vi "Emballage mail expedition.vi"(1 "Tableau mail expedition":string[][](array[string]), 2 "Article":string) -> (0 "Email expedition":string)   [LabVIEW 2020]
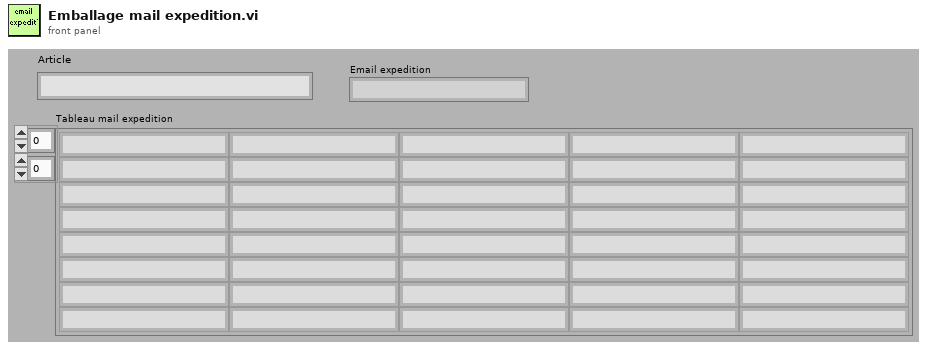
[diagram p1: front panel]
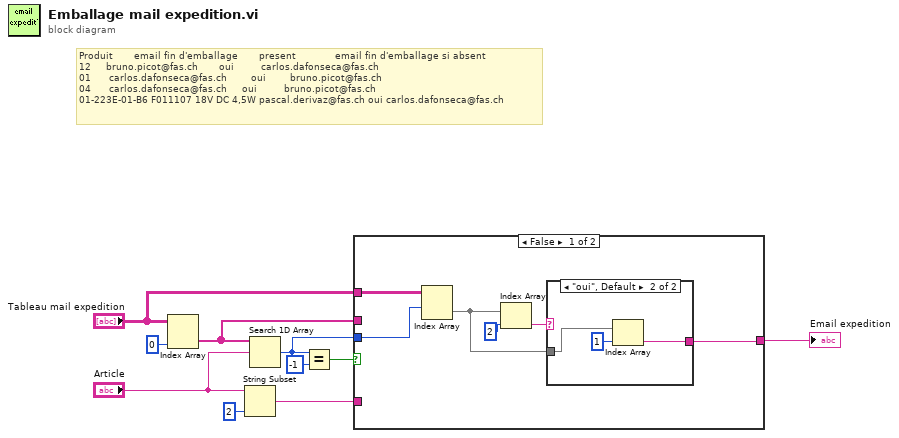
[diagram p0: block diagram]
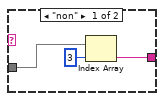
[diagram p2: hidden frame]
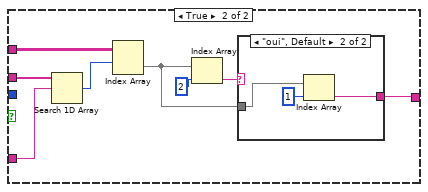
[diagram p3: hidden frame]
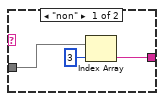
[diagram p4: hidden frame]
diagram:
  # "Produit\t      email fin d'emballage\t      present\t            email fin d'emballage si absent\n12     bruno.picot@fas.ch\t      oui\t        carlos.dafonseca@fas.ch\t\n01\t     carlos.dafonseca@fas.ch\t       oui\t       bruno.picot@fas.ch\n04\t     carlos.dafonseca@fas.ch\t    oui\t        bruno.picot@fas.ch\n01-223E-01-B6 F011107 18V DC 4,5W\tpascal.derivaz@fas.ch\toui\tcarlos.dafonseca@fas.ch"
  n1 = Index Array(array="Tableau mail expedition", index (col)=0 ("indice désactivé (col)")) -> (element=w4:string[])  [unwired: 1 in]
  n2 = String Subset(string="Article", length (rest)=2 ("longueur (reste)")) -> (substring=w5:string)  [unwired: 1 in]
  n3 = Search 1D Array(1D array=w4, element="Article") -> (index of element=w1:i32)  [unwired: 1 in]
  n4 = Equal?(x=w1, y=-1) -> (x = y?=w8:bool)
  n5 = case shown="False" w8 {
    tunnel: w5 -> [_ w30]
    tunnel: w4 -> [_ w29]
    tunnel: "Tableau mail expedition" -> [w12 w28]
    tunnel: [w13 w23] -> w2
    tunnel: w1 -> [w11 _]
    frame False {
      n6 = Index Array(array=w12, index (row)=w11) -> (element=w14:string[])  [unwired: 1 in]
      n7 = Index Array(array=w14, index=2 ("indice")) -> (element=w15:string)
      n8 = case shown="\"oui\", Default" w15 {
        tunnel: w14 -> [w18 w22]
        tunnel: [w17 w20] -> w13
        frame "non" {
          n9 = Index Array(array=w18, index=3 ("indice")) -> (element=w17:string)
        }
        frame "oui", Default {
          n10 = Index Array(array=w22, index=1 ("indice")) -> (element=w20:string)
        }
      }
    }
    frame True {
      n11 = Search 1D Array(1D array=w29, element=w30) -> (index of element=w27:i32)  [unwired: 1 in]
      n12 = Index Array(array=w28, index (row)=w27) -> (element=w24:string[])  [unwired: 1 in]
      n13 = Index Array(array=w24, index=2 ("indice")) -> (element=w25:string)
      n14 = case shown="\"oui\", Default" w25 {
        tunnel: w24 -> [w32 w36]
        tunnel: [w31 w34] -> w23
        frame "non" {
          n15 = Index Array(array=w32, index=3 ("indice")) -> (element=w31:string)
        }
        frame "oui", Default {
          n16 = Index Array(array=w36, index=1 ("indice")) -> (element=w34:string)
        }
      }
    }
  }
  "Email expedition" <- w2
